vi "export labview dosctrings.vi"() -> ()   [LabVIEW 2020]
uses:
  <vilib>/xml/NI_XML.lvlib
  <vilib>/xml/Load XML File.vi
  <vilib>/xml/Close Reference(Node).vi
panel:
  out "error out":errorcluster
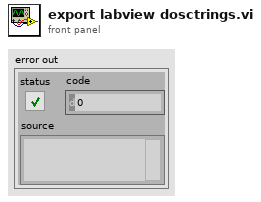
[diagram p1: front panel]
types:
  T1 = cluster{"name":string, "palette node":refnum<k20>, "parent":i32}[]
  T2 = cluster{"owning palette":cluster{"name":string, "palette node":refnum<k20>, "parent":i32}, "items":cluster{"name":string, "path":path, "node":refnum<k20>}[]}[]
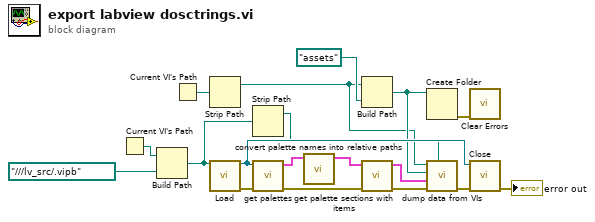
[diagram p0: block diagram]
diagram:
  n1 = Current VI's Path() -> (path=w18:path)
  n2 = Build Path(base path=w18, name or relative path=path "../../../lv_src/.vipb") -> (appended path=w2:path)
  n3 = Current VI's Path() -> (path=w10:path)
  n4 = Strip Path(path=w10) -> (stripped path=w6:path)  [unwired: 1 out]
  n5 = call-poly <vilib>:"Load.vi"("path to XML document"=w2) -> ("DOM document out"=w15:refnum<k20>, "error out"=w16:errorcluster)  [unwired: 12 in, 1 out]
  n6 = Strip Path(path=w2) -> (stripped path=w1:path)  [unwired: 1 out]
  n7 = call "get palettes.vi"("error in (no error)"=w16, "Refnum in"=w15) -> ("error out"=w13:errorcluster, "palettes"=w14:T1)  [unwired: 8 in]
  n8 = call "convert palette names into relative paths.vi"("palettes"=w14) -> ("nested palettes"=w12:T1)  [unwired: 10 in]
  n9 = Build Path(base path=w6, name or relative path=path "assets") -> (appended path=w7:path)
  n10 = call "get palette sections with items.vi"("error in (no error)"=w13, "nested palettes"=w12) -> ("error out"=w5:errorcluster, "palette sections"=w11:T2)  [unwired: 8 in]
  n11 = Create Folder(path (use dialog)=w7) -> (error out=w8:errorcluster)  [unwired: 2 in, 2 out]
  n12 = call "dump data from VIs.vi"("vipb base"=w1, "error in (no error)"=w5, "palette sections"=w11, "assets"=w7, "docs folder"=w6) -> ("error out"=w4:errorcluster)  [unwired: 6 in]
  n13 = call <vilib>:"Clear Errors.vi"("error in (no error)"=w8) -> ()  [unwired: 5 in, 2 out]
  n14 = call-poly <vilib>:"Close.vi"("error in (no error)"=w4, "node"=w15) -> ("error out"=→"error out":errorcluster)  [unwired: 7 in]
